vi "read_params.vi"(8 "error in (no error)":errorcluster, 11 "StackingClassifier in":refnum<class "StackingClassifier.lvclass">) -> (0 "error out":errorcluster, 2 "params":T1={"estimators"=[], "cv"=5.0, "stack_method"="auto", "n_jobs"=1.0, "passthrough"=FALSE, "verbose"=0.0}, 3 "StackingClassifier out":refnum<class "StackingClassifier.lvclass">)   [LabVIEW 2020, in "StackingClassifier.lvclass"]
uses:
  StackingClassifier.lvclass
  Controls/stacking_classifier_params.ctl
  StackingClassifier.lvclass/StackingClassifier.ctl
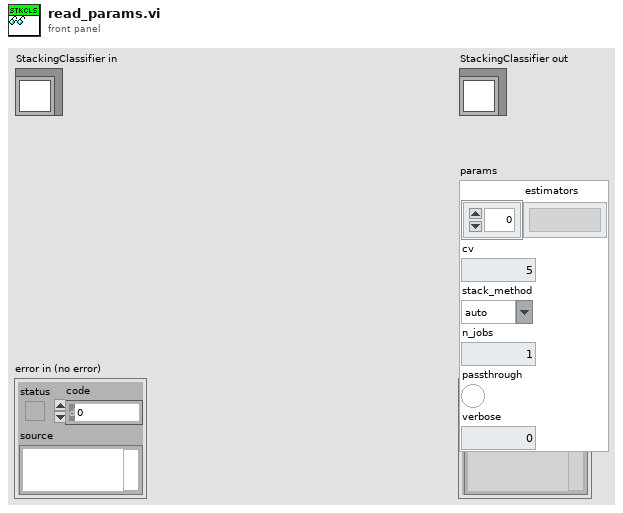
[diagram p1: front panel]
types:
  T1 = typedef "stacking_classifier_params.ctl" = cluster{"estimators":string[], "cv":dbl, "stack_method":string, "n_jobs":dbl, "passthrough":bool, "verbose":dbl}
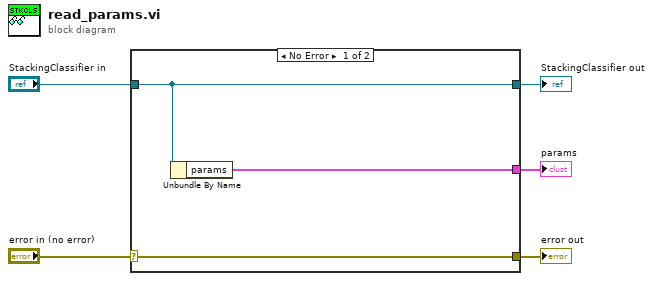
[diagram p0: block diagram]
diagram:
  n1 = case shown="No Error" "error in (no error)" {
    selector: "error in (no error)" -> [w8 w9]
    tunnel: [w8 w9] -> w4
    tunnel: [w7 w10] -> w2
    tunnel: "StackingClassifier in" -> [w7 w10]
    tunnel: [w6 _] -> w1
    frame No Error {
      n2 = Unbundle By Name(w7) -> ("params"=w6:T1)
    }
    frame Error {
    }
  }
  "error out" <- w4
  "StackingClassifier out" <- w2
  "params" <- w1
